vi "histogram3_image.vi"() -> ()   [LabVIEW 2020]
uses:
  <vilib>/vision/NI_Vision_Development_Module.lvlib
panel:
  out "색상":T1(ring)
  out "색숫자":u32
  in  "File Path":path
  out "히스토그램2":u8[][](graph)
  out "Image Out":T2(plugin-control)
  in  "캡쳐":bool
  in  "정지":bool
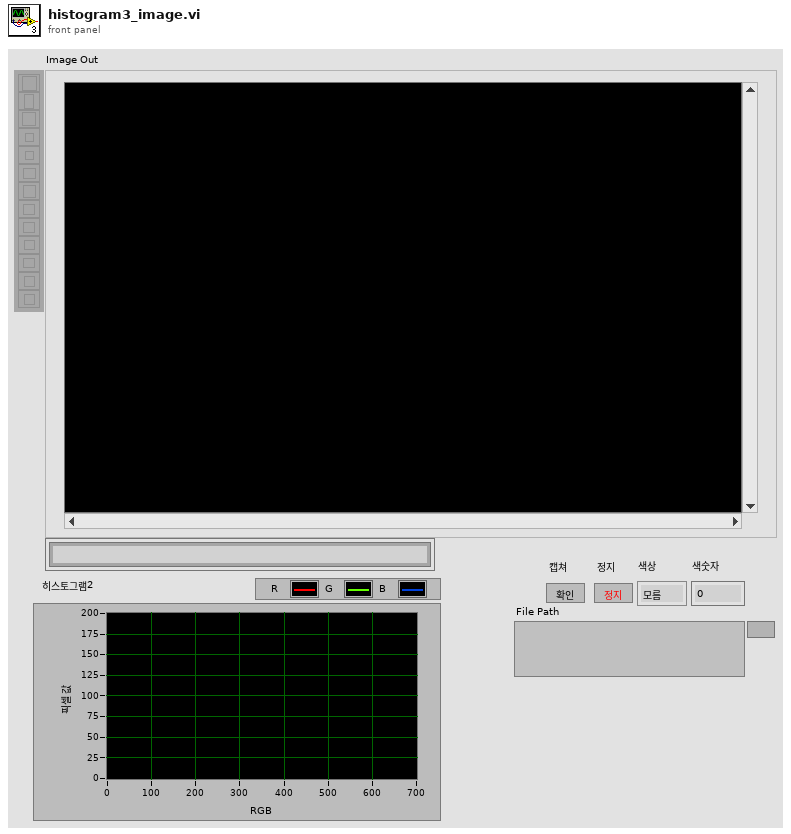
[diagram p1: front panel]
types:
  T1 = enum16{"모름", "빨강", "녹색", "노랑", "파랑", "보라", "하늘", "흰색"}
  T2 = typedef "IMAQ Image.ctl" = refnum<image>
  T3 = enum16{"모름", "빨강", "녹색", "노랑", "파랑", "보라", "하늘", "흰색"}[]
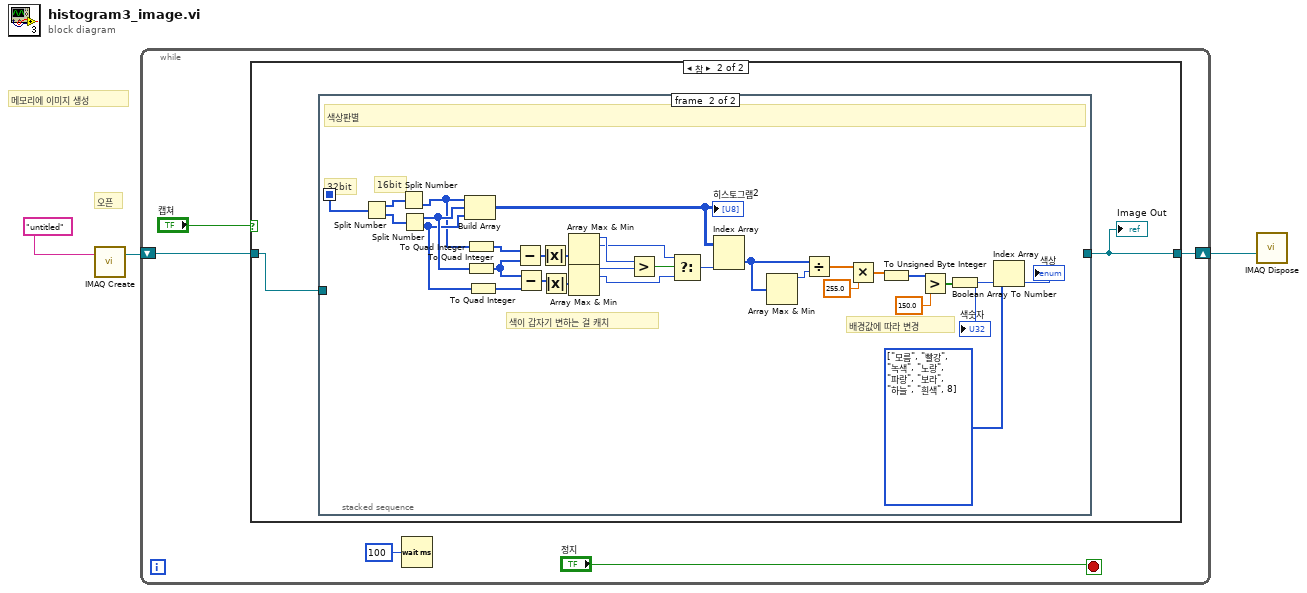
[diagram p0: block diagram]
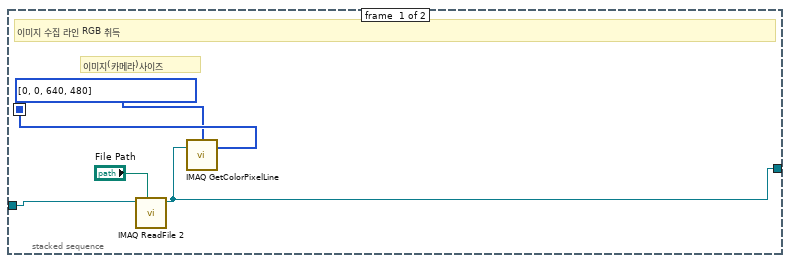
[diagram p3: hidden frame]
diagram:
  # "오픈"
  # "메모리에 이미지 생성"
  n1 = call "IMAQ Create"("Image Name"="untitled") -> ("New Image"=w2:T2)  [unwired: 4 in, 1 out]
  n2 = while {
    shift-right: [w7] -> w1
    shift-left: w2 -> [w8]
    stop <- "정지" stop-if-true
    n3 = case shown="참" "캡쳐" {
      tunnel: w8 -> [w9 w11]
      tunnel: [w9 w10] -> w7
      frame False {
      }
      frame True {
        n4 = stacked-sequence {
          seq-local: [w16 _] -> [_ w47]
          tunnel: w11 -> [w14 _]
          tunnel: [w12 _] -> w10
          frame #0 {
            # "이미지(카메라)사이즈"
            # "이미지 수집 라인 RGB 취득"
            n5 = call "IMAQ ReadFile 2"("File Path"="File Path", "Image"=w14) -> ("Image Out"=w12:T2)  [unwired: 5 in, 4 out]
            n6 = call "IMAQ GetColorPixelLine"("Line Coordinates"=i32[] [0, 0, 640, 480], "Image"=w12) -> ("Pixels Line (U32)"=w16:u32[])  [unwired: 2 in, 2 out]
          }
          frame #1 {
            w19 = T3 [enum."모름", enum."빨강", enum."녹색", enum."노랑", enum."파랑", enum."보라", enum."하늘", enum."흰색", 8] items=["모름", "빨강", "녹색", "노랑", "파랑", "보라", "하늘", "흰색"] ("배열")
            # "배경값에 따라 변경"
            # "색이 갑자기 변하는 걸 캐치"
            # "16bit"
            # "32bit"
            # "색상판별"
            n7 = Split Number(x=w47) -> (hi(x)=w46:u16[], lo(x)=w45:u16[])
            n8 = Split Number(x=w46) -> (lo(x)=w42:u8[])  [unwired: 1 out]
            n9 = Split Number(x=w45) -> (hi(x)=w44:u8[], lo(x)=w43:u8[])
            n10 = Build Array(w42, w44, w43) -> (w33:u8[][])
            "히스토그램2" <- w33
            n11 = To Quad Integer(1:w42) -> (0:w41:i64[])
            n12 = To Quad Integer(1:w44) -> (0:w40:i64[])
            n13 = To Quad Integer(1:w43) -> (0:w39:i64[])
            n14 = Subtract(x=w41, y=w40) -> (x-y=w31:i64[])
            n15 = Subtract(x=w40, y=w39) -> (x-y=w30:i64[])
            n16 = Absolute Value(x=w31) -> (abs(x)=w29:i64[])
            n17 = Absolute Value(x=w30) -> (abs(x)=w28:i64[])
            n18 = Array Max & Min(array=w29) -> (max value=w38:i64, max index (indices)=w35:i32)  [unwired: 2 out]
            n19 = Array Max & Min(array=w28) -> (max value=w37:i64, max index (indices)=w34:i32)  [unwired: 2 out]
            n20 = Greater?(x=w38, y=w37) -> (0:w36:bool)
            n21 = Select(t=w35, s=w36, f=w34) -> (s? t:f=w32:i32)
            n22 = Index Array(array=w33, index (col)=w32) -> (element=w26:u8[])  [unwired: 1 in]
            n23 = Array Max & Min(array=w26) -> (max value=w27:u8)  [unwired: 3 out]
            n24 = Divide(x=w26, y=w27) -> (x/y=w25:dbl[])
            n25 = Multiply(x=w25, y=255.0) -> (x*y=w17:dbl[])
            n26 = To Unsigned Byte Integer(number=w17) -> (unsigned 8bit integer=w23:u8[])
            n27 = Greater?(x=w23, y=150.0) -> (0:w21:bool[])
            n28 = Boolean Array To Number(Boolean array=w21) -> (number=w20:u32)
            "색숫자" <- w20
            n29 = Index Array(array=w19, index=w20) -> (element=→"색상":T1)
          }
        }
        "Image Out" <- w10
      }
    }
    n30 = Wait (ms)(milliseconds to wait=u32 100 ("대기 시간 (ms)")) -> ()  [unwired: 1 out]
  }
  n31 = call "IMAQ Dispose"("Image"=w1) -> ()  [unwired: 5 in, 1 out]
